vi "OAT Torsional Vibration (Analog Tacho).vi"   [LabVIEW 2017, in "SoundVib_Torsional.lvlib"]
doc: "Calculates torsional vibration signals from analog tachometer signals. This VI can return torsional vibration signals as either waveform signals or even-angle signals. Wire data to the <B>analog tacho signal</B> input to determine the polymorphic instance to use or manually select the instance."
uses:
  <vilib>/addons/Sound and Vibration/Order Analysis/Torsional Vibration/SoundVib_Torsional.lvlib
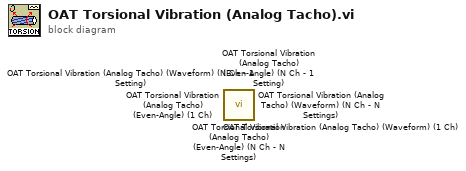
[diagram p0: block diagram]
diagram:
  n1 = call <vilib>:"OAT Torsional Vibration (Analog Tacho) (Even-Angle) (N Ch - N Settings).vi"() -> ()  [unwired: 14 in, 6 out]
  n2 = call <vilib>:"OAT Torsional Vibration (Analog Tacho) (Even-Angle) (N Ch - 1 Setting).vi"() -> ()  [unwired: 14 in, 6 out]
  n3 = call <vilib>:"OAT Torsional Vibration (Analog Tacho) (Even-Angle) (1 Ch).vi"() -> ()  [unwired: 14 in, 6 out]
  n4 = call <vilib>:"OAT Torsional Vibration (Analog Tacho) (Waveform) (N Ch - N Settings).vi"() -> ()  [unwired: 16 in, 4 out]
  n5 = call <vilib>:"OAT Torsional Vibration (Analog Tacho) (Waveform) (N Ch - 1 Setting).vi"() -> ()  [unwired: 16 in, 4 out]
  n6 = call <vilib>:"OAT Torsional Vibration (Analog Tacho) (Waveform) (1 Ch).vi"() -> ()  [unwired: 16 in, 4 out]
